vi "ProbabilityDensity.vi"(9 "grid y":dbl format="%#_13g", 10 "grid x":dbl format="%#_13g", 11 "IA state":T1={"our_robots"=[], "enemy_robots"=[], "balls"=[], "geometry"={"line_width"=0, "field_length"=0, "field_width"=0, "boundary_width"=0, "referee_width"=0, "goal_width"=0, "goal_depth"=0, "goal_wall_width"=0, "center_circle_radius"=0, "defense_radius"=0, "defense_stretch"=0, "free_kick_from_defense_dist"=0, "penalty_spot_from_field_line_dist"=0, "penalty_line_from_spot_dist"=0}, "IA Judge"={"stage"="", "command"="", "our_goalie_id"=0.0, "enemy_goalie_id"=0.0, "command enum"=enum."Halt", "Time"=enum."Azul"}, "Received Timestamp"=timestamp(0 s since 1904-01-01), "Events"={"Touch"=FALSE, "Ball out"=FALSE, "id touch"=0.0, "Ball out of \nVision"=FALSE, "Ball inside \nGoalie area"=FALSE, "Robot not responding"=FALSE, "Robots responding status"=[1.0, 1.0, 1.0, 1.0, 1.0, 1.0], "Enemy Ball \nPossession"=FALSE, "Pass State"=FALSE, "id end of pass"=0.0, "Kick"=FALSE, "Id ini Possession"=0.0, "Ball Possesion"=FALSE, "Id Possesion"=0.0}}) -> (0 "grid y out":dbl format="%#_13g", 1 "grid x out":dbl format="%#_13g", 2 "3D Probability Matrix":dbl[][][](array[numeric]))   [LabVIEW 2017]
uses:
  Core/AI Input.ctl
  Core/AI Robot.ctl
  Intel/Functions Enum.ctl
  Intel/AttackerStates.ctl
  Core/AI Ball.ctl
  Core/Field Size.ctl
  Core/AI Judge.ctl
  Intel/Command Enum.ctl
  Util/Events/Events.ctl
panel:
  out "error out":errorcluster
  out "path out":path
  in  "error in":errorcluster
  in  "path in":path
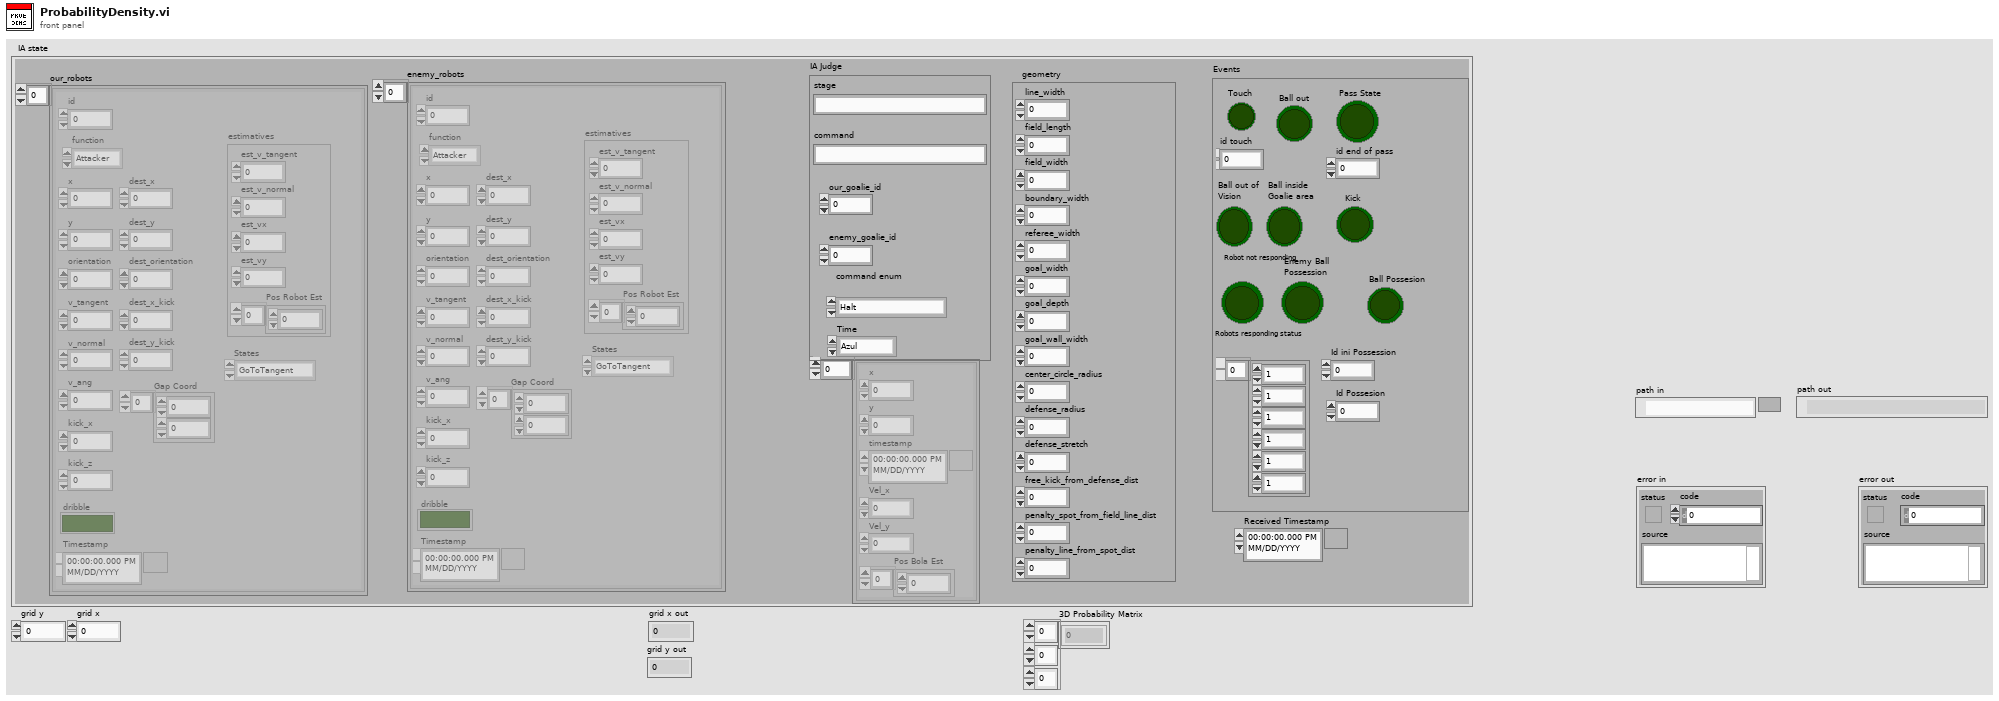
[diagram p1: front panel]
types:
  T1 = typedef "AI Input.ctl" = cluster{"our_robots":T2[], "enemy_robots":T2[], "balls":T5[], "geometry":T6, "IA Judge":T7, "Received Timestamp":timestamp, "Events":T9}
  T2 = typedef "AI Robot.ctl" = cluster{"id":u32, "function":T3, "x":dbl, "y":dbl, "orientation":dbl, "v_tangent":dbl, "v_normal":dbl, "v_ang":dbl, "kick_x":dbl, "kick_z":dbl, "dribble":bool, "Timestamp":timestamp, "dest_x":dbl, "dest_y":dbl, "dest_orientation":dbl, "estimatives":cluster{"est_v_tangent":dbl, "est_v_normal":dbl, "est_vx":dbl, "est_vy":dbl, "Pos Robot Est":dbl[]}, "dest_x_kick":dbl, "dest_y_kick":dbl, "Gap Coord":dbl[], "States":T4}
  T3 = typedef "Functions Enum.ctl" = enum16{"Attacker", "Goalie", "Defender", "Striker", "Goto 0", "Dummy", "Kicker", "ZigZag"}
  T4 = typedef "AttackerStates.ctl" = enum16{"Pass", "GoToTangent", "BallGetting", "GoToKick", ""}
  T5 = typedef "AI Ball.ctl" = cluster{"x":dbl, "y":dbl, "timestamp":timestamp, "Vel_x":dbl, "Vel_y":dbl, "Pos Bola Est":dbl[]}
  T6 = typedef "Field Size.ctl" = cluster{"line_width":u32, "field_length":u32, "field_width":u32, "boundary_width":u32, "referee_width":u32, "goal_width":u32, "goal_depth":u32, "goal_wall_width":u32, "center_circle_radius":u32, "defense_radius":u32, "defense_stretch":u32, "free_kick_from_defense_dist":u32, "penalty_spot_from_field_line_dist":u32, "penalty_line_from_spot_dist":u32}
  T7 = typedef "AI Judge.ctl" = cluster{"stage":string, "command":string, "our_goalie_id":dbl, "enemy_goalie_id":dbl, "command enum":T8, "Time":enum16{"Azul", "Amarelo"}}
  T8 = typedef "Command Enum.ctl" = enum16{"Halt", "Stop", "Force Start", "PKA Normal Start", "Prepare Kickoff Ally", "PKE Normal Start", "Prepare Kickoff Enemy", "Prepare Penalty Ally", "PPA Normal Start", "Prepare Penalty Enemy", "PPE Normal Start", "Direct Free Enemy", "Direct Free Ally", "Indirect Free Enemy", "Indirect Free Ally", "Timeout Enemy", "Timeout Ally", "Goal Enemy", "Goal Ally", "Ball Placement Enemy", "Ball Placement Ally", "Normal Half Time", "Extra Time Break", "Extra Half Time", "None", "Post Game"}
  T9 = typedef "Events.ctl" = cluster{"Touch":bool, "Ball out":bool, "id touch":dbl, "Ball out of \nVision":bool, "Ball inside \nGoalie area":bool, "Robot not responding":bool, "Robots responding status":dbl[], "Enemy Ball \nPossession":bool, "Pass State":bool, "id end of pass":dbl, "Kick":bool, "Id ini Possession":dbl, "Ball Possesion":bool, "Id Possesion":dbl}
  T10 = enum16{"open", "replace", "create", "open or create", "replace or create", "replace or create with confirmation"}
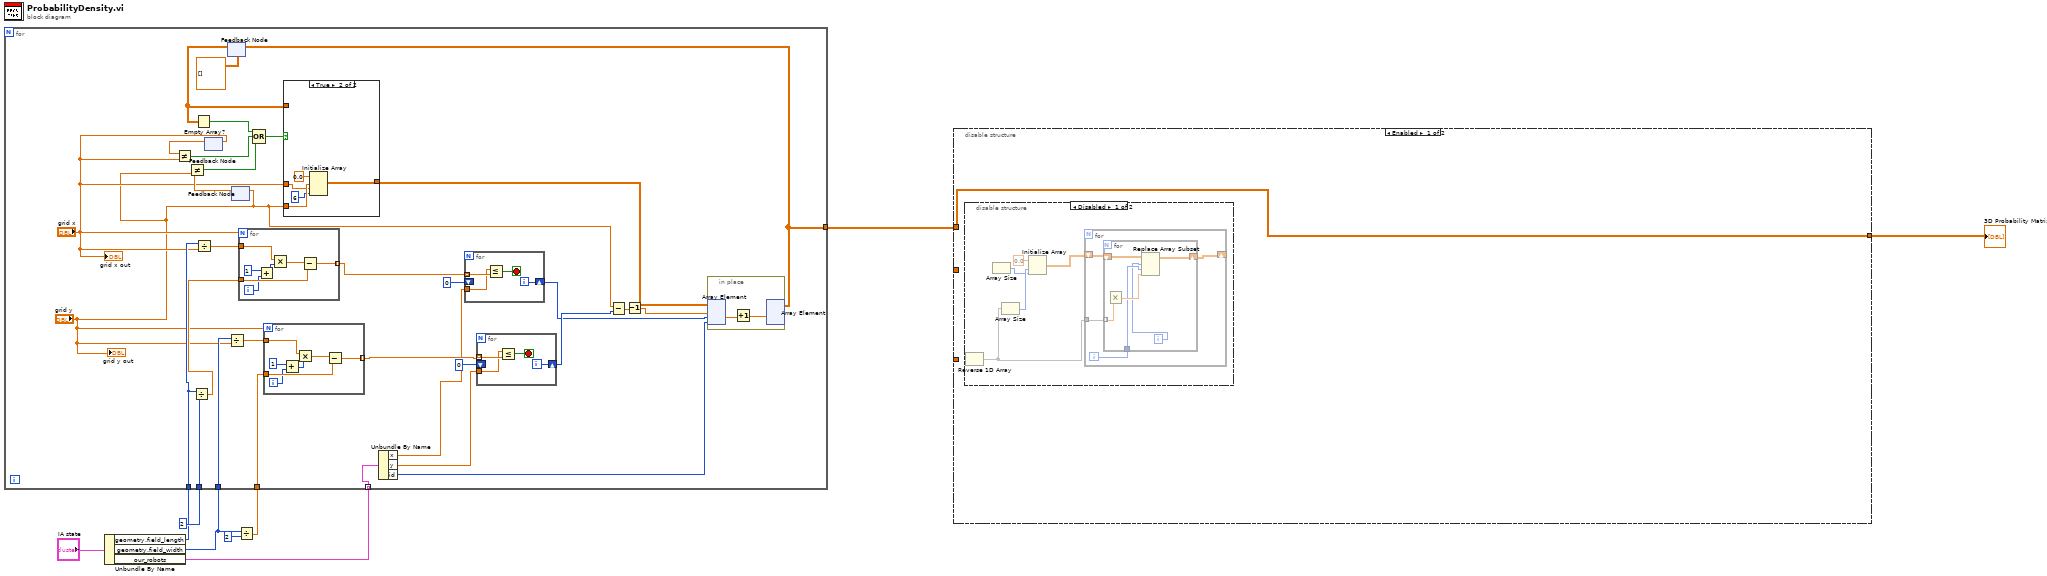
[diagram p0: block diagram]
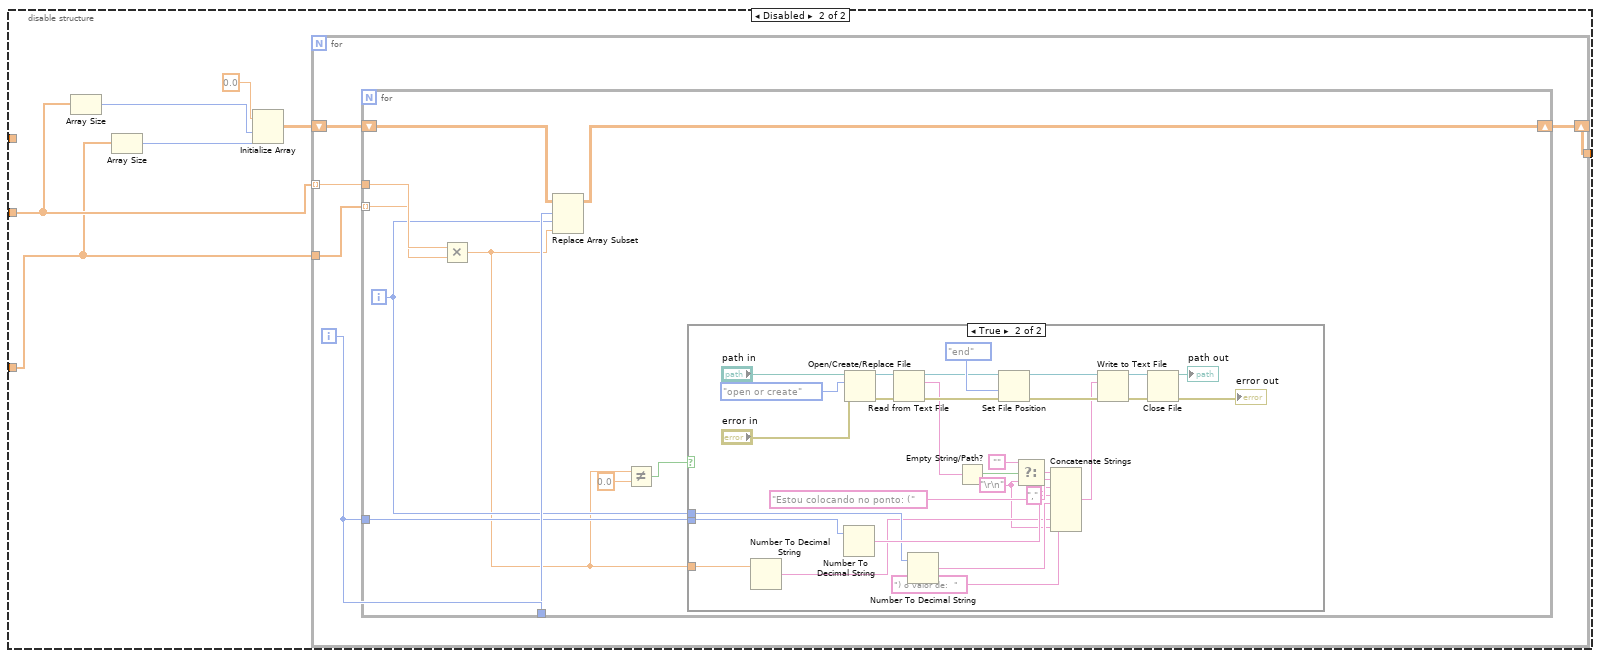
[diagram p4: hidden frame]
diagram:
  n1 = Unbundle By Name("IA state") -> ("geometry.field_length"=w5:u32, "geometry.field_width"=w4:u32, "our_robots"=w2:T2[])
  n2 = Divide(x=w4, y=u32 2) -> (x/y=w6:dbl)
  n3 = for {
    tunnel: u32 2 ("y") -> [w30]
    tunnel: w6 -> [w28]
    tunnel: w5 -> [w27]
    tunnel: w4 -> [w26]
    tunnel: [w19] -> w3
    tunnel: w2 -> [w11] mode=indexing
    n4 = Divide(x=w27, y=w30) -> (x/y=w29:dbl)
    n5 = Divide(x=w27, y="grid x") -> (x/y=w40:dbl)
    n6 = feedback #1() -> (w39:dbl)  [unwired: 1 in]
    n7 = Not Equal?(x=w39, y="grid x") -> (x != y?=w36:bool)
    n8 = feedback-in #1("grid x") -> ()
    n9 = feedback #2(dbl[][][] []) -> (w33:dbl[][][])
    n10 = Empty Array?(array=w33) -> (empty?=w37:bool)
    n11 = Divide(x=w26, y="grid y") -> (x/y=w25:dbl)
    n12 = feedback #3() -> (w38:dbl)  [unwired: 1 in]
    n13 = Not Equal?(x=w38, y="grid y") -> (x != y?=w35:bool)
    n14 = feedback-in #3("grid y") -> ()
    n15 = for {
      N: "grid x" -> [_]
      tunnel: w40 -> [w70]
      tunnel: w29 -> [w67]
      tunnel: [w68] -> w23 mode=indexing
      i -> [w66]
      n16 = Add(x=1, y=w66) -> (x+y=w64:i32)
      n17 = Multiply(x=w70, y=w64) -> (x*y=w69:dbl)
      n18 = Subtract(x=w69, y=w67) -> (x-y=w68:dbl)
    }
    n19 = Compound Arithmetic op=OR(w37, w36, w35) -> (w34:bool)
    n20 = for {
      N: "grid y" -> [_]
      tunnel: w25 -> [w63]
      tunnel: w28 -> [w60]
      tunnel: [w61] -> w24 mode=indexing
      i -> [w59]
      n21 = Add(x=1, y=w59) -> (x+y=w58:i32)
      n22 = Multiply(x=w63, y=w58) -> (x*y=w62:dbl)
      n23 = Subtract(x=w62, y=w60) -> (x-y=w61:dbl)
    }
    n24 = case shown="True" w34 {
      tunnel: "grid x" -> [_ w53]
      tunnel: "grid y" -> [_ w54]
      tunnel: w33 -> [w51 _]
      tunnel: [w51 w55] -> w21
      frame False {
      }
      frame True {
        n25 = Initialize Array(0.0 ("element"), w54, w53, 6 ("dimension size")) -> (w55:dbl[][][])
      }
    }
    n26 = Unbundle By Name(w11) -> ("x"=w13:dbl, "y"=w12:dbl, "id"=w10:u32)
    n27 = for {
      shift-right: [w49] -> w16
      shift-left: 0 -> [_]
      tunnel: w23 -> [w48] mode=indexing
      tunnel: w13 -> [w47]
      i -> [w49]
      stop <- w50 stop-if-true
      n28 = Less Or Equal?(x=w47, y=w48) -> (x <= y?=w50:bool)
    }
    n29 = for {
      shift-right: [w45] -> w17
      shift-left: 0 -> [_]
      tunnel: w24 -> [w44] mode=indexing
      tunnel: w12 -> [w43]
      i -> [w45]
      stop <- w46 stop-if-true
      n30 = Less Or Equal?(x=w43, y=w44) -> (x <= y?=w46:bool)
    }
    n31 = Subtract(x="grid y", y=w17) -> (x-y=w15:dbl)
    n32 = Decrement(x=w15) -> (x-1=w14:dbl)
    n33 = in-place {
      n34 = in-place-array #4(w21, w14, w16, w10) -> (w42:dbl)
      n35 = Increment(x=w42) -> (x+1=w41:dbl)
      n36 = in-place-array #4(w41) -> (w19:dbl[][][])  [unwired: 3 out]
    }
    n37 = feedback-in #2(w19) -> ()
    "grid x out" <- "grid x"
    "grid y out" <- "grid y"
  }
  n38 = disable-structure shown="Enabled" {
    disable-tunnel: _ -> [_ w91]
    disable-tunnel: _ -> [_ w93]
    disable-tunnel: [w71 w87] -> w1
    disable-tunnel: w3 -> [w71 _]
    frame Enabled {
      n39 = disable-structure shown="Disabled" {
        frame Disabled {
          n40 = Reverse 1D Array() -> (reversed array=w72:dbl[])  [unwired: 1 in]
          n41 = Array Size() -> (size(s)=w73:i32)  [unwired: 1 in]
          n42 = Array Size(array=w72) -> (size(s)=w74:i32)
          n43 = Initialize Array(0.0 ("element"), w74, w73) -> (w75:dbl[][])
          n44 = for {
            tunnel: w72 -> [w80]
            shift-right: [w77] -> _
            shift-left: w75 -> [w79]
            i -> [w78]
            n45 = for {
              tunnel: w80 -> [w85] mode=indexing
              tunnel: w78 -> [w82]
              shift-right: [w83] -> w77
              shift-left: w79 -> [w86]
              i -> [w81]
              n46 = Multiply(y=w85) -> (x*y=w84:dbl)  [unwired: 1 in]
              n47 = Replace Array Subset(array=w86, new element=w84, index (row)=w81, index (col)=w82) -> (w83:dbl[][])
            }
          }
        }
        frame Enabled {
        }
      }
    }
    frame Disabled {
      n48 = Array Size(array=w93) -> (size(s)=w92:i32)
      n49 = Array Size(array=w91) -> (size(s)=w90:i32)
      n50 = Initialize Array(0.0 ("element"), w92, w90) -> (w88:dbl[][])
      n51 = for {
        tunnel: w93 -> [w98] mode=indexing
        tunnel: w91 -> [w97]
        shift-right: [w95] -> w87
        shift-left: w88 -> [w96]
        i -> [w94]
        n52 = for {
          tunnel: w98 -> [w106]
          tunnel: w97 -> [w105] mode=indexing
          tunnel: w94 -> [w107]
          shift-right: [w104] -> w95
          shift-left: w96 -> [w108]
          tunnel: w94 -> [w103]
          i -> [w102]
          n53 = Multiply(x=w106, y=w105) -> (x*y=w101:dbl)
          n54 = Replace Array Subset(array=w108, new element=w101, index (row)=w107, index (col)=w102) -> (w104:dbl[][])
          n55 = Not Equal?(x=w101, y=0.0) -> (x != y?=w99:bool)
          n56 = case shown="True" w99 {
            tunnel: w103 -> [_ w117]
            tunnel: w102 -> [_ w114]
            tunnel: w101 -> [_ w111]
            frame False {
            }
            frame True {
              w109 = "\r\n"
              n57 = Number To Decimal String(number=w111) -> (decimal integer string=w110:string)  [unwired: 1 in]
              n58 = Number To Decimal String(number=w117) -> (decimal integer string=w116:string)  [unwired: 1 in]
              n59 = Open/Create/Replace File(file path (use dialog)="path in", error in="error in", operation (0:open)=T10."open or create") -> (refnum out=w134:refnum<file>, error out=w133:errorcluster)  [unwired: 3 in, 1 out]
              n60 = Read from Text File(file (use dialog)=w134, error in=w133) -> (refnum out=w128:refnum<file>, text=w122:string, error out=w130:errorcluster)  [unwired: 2 in, 1 out]
              n61 = Number To Decimal String(number=w114) -> (decimal integer string=w113:string)  [unwired: 1 in]
              n62 = Empty String/Path?(string/path=w122) -> (empty?=w129:bool)
              n63 = Set File Position(refnum=w128, from (0:start)=enum16{"start", "end", "current"}."end", error in=w130) -> (refnum out=w127:refnum<file>, error out=w126:errorcluster)  [unwired: 1 in]
              n64 = Select(t="", s=w129, f=w109) -> (s? t:f=w125:string)
              n65 = Concatenate Strings(w125, "Estou colocando no ponto: (" ("string"), w116, "," ("string"), w113, ") o valor de:  " ("string"), w110, w109) -> (w124:string)
              n66 = Write to Text File(file (use dialog)=w127, text=w124, error in=w126) -> (refnum out=w136:refnum<file>, error out=w135:errorcluster)  [unwired: 1 in, 1 out]
              n67 = Close File(refnum=w136, error in=w135) -> (path=→"path out":path, error out=→"error out":errorcluster)
            }
          }
        }
      }
    }
  }
  "3D Probability Matrix" <- w1
